vi "Keep position above object.vi"(8 "bottom":dbl, 9 "right":dbl, 10 "top":dbl, 11 "left":dbl) -> (0 "Hover":bool, 1 "Roll":dbl, 2 "Pitch":dbl)   [LabVIEW 2014]
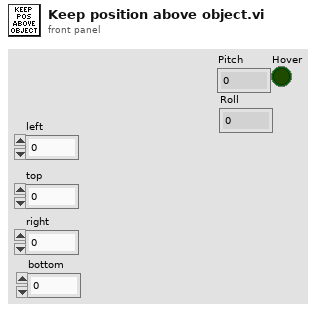
[diagram p1: front panel]
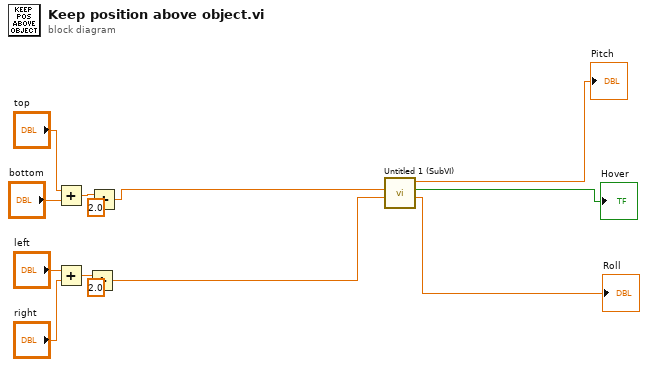
[diagram p0: block diagram]
diagram:
  n1 = Add(x="top", y="bottom") -> (x+y=w7:dbl)
  n2 = Add(x="left", y="right") -> (x+y=w6:dbl)
  n3 = Divide(x=w6, y=2.0) -> (x/y=w4:dbl)
  n4 = Divide(x=w7, y=2.0) -> (x/y=w5:dbl)
  n5 = call "Untitled 1 (SubVI).vi"("X"=w4, "Y"=w5) -> ("Roll"=→"Roll":dbl, "Hover"=→"Hover":bool, "Pitch"=→"Pitch":dbl)  [unwired: 7 in]
